vi "LINC Register Packet.vi"(4 "alternate data names (empty)":string[](array[string]), 5 "ID":i32=-1, 6 "alternate packet names (empty)":string[](array[string]), 7 "single packet (F)":bool, 8 "error in (no error)":errorcluster, 9 "type (CMD)":enum16{"CMD", "TLM", "CMD_HDR", "TLM_HDR"}(ring), 10 "controls":refnum<vi>[](array[refnum]), 11 "LINC session":refnum<class "LINC.lvclass">) -> (0 "error out":errorcluster, 3 "dup LINC session":refnum<class "LINC.lvclass">)   [LabVIEW 2018, in "STEPkgDriver_LINC.lvlib" / "LINC.lvclass"]
uses:
  LINC.lvclass
  STEPkgDriver_LINC.lvlib
  LINC Global Mode.ctl
  LINC Config.ctl
  LINC Global Config Mode.ctl
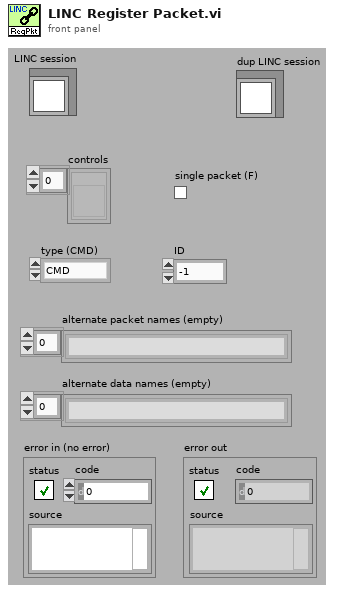
[diagram p1: front panel]
types:
  T1 = typedef "STEPkgDriver_LINC.lvlib/LINC Global Config Mode.ctl" = enum16{"INIT", "CLEAR", "SET_CMD_CB", "SET_TLM_CB", "SET_CMD_FIELDS", "SET_TLM_FIELDS", "SET_ID", "GET_CONFIG"}
  T2 = typedef "STEPkgDriver_LINC.lvlib/LINC Config.ctl" = cluster{"cmd callback":refnum<vi>, "tlm callback":refnum<vi>, "cmd ID bitoffset":i32, "cmd ID bitsize":i32, "cmd IDs":i32[], "tlm ID bitoffset":i32, "tlm ID bitsize":i32, "tlm IDs":i32[], "cmd header fields":i32, "tlm header fields":i32, "tlm header size":i32}
  T3 = typedef "STEPkgDriver_LINC.lvlib/LINC Global Mode.ctl" = enum16{"INIT", "CLEAR", "ADD_PKT_HDR", "ADD_PKT", "GET_PKT_NAMES", "GET_PKT_DESC", "GET_PKT_HDR", "GET_PKT", "SET_PKT", "SET_DATA", "SIM_EN", "SIM_DS"}
  T4 = typedef "STEPkgDriver_LINC.lvlib/LINC Format Prototype.ctl" = cluster{"type":string, "bit offset":i32, "bit size":i32, "format":string, "unit":string, "description":string, "state values":i64[], "states":string[], "max":string, "min":string, "default":string, "array":bool, "bit element size":i32, "poly bound":dbl[], "poly scale":cluster{"coefficients":dbl[]}[], "labview size":i32, "simulate":bool, "ID":bool, "required":bool}
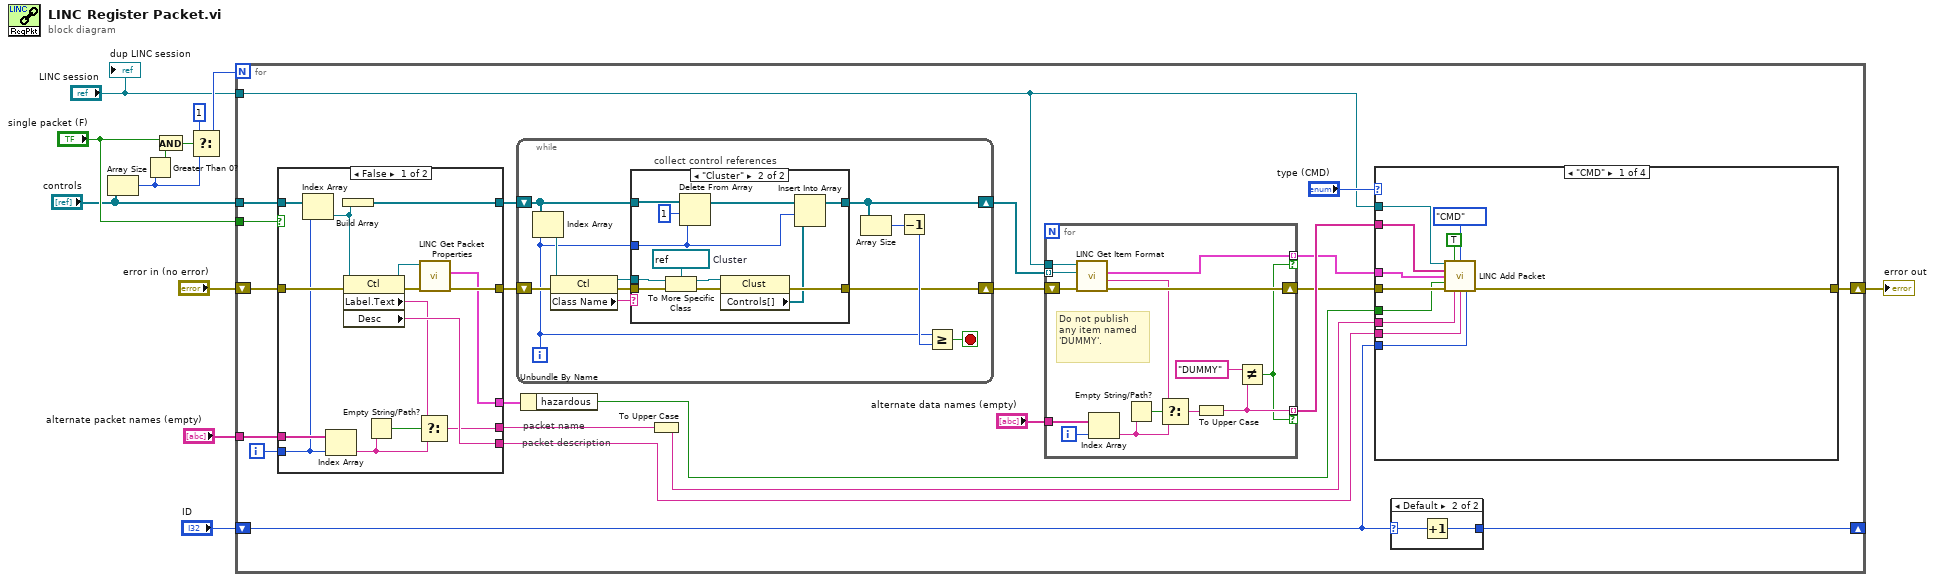
[diagram p0: block diagram]
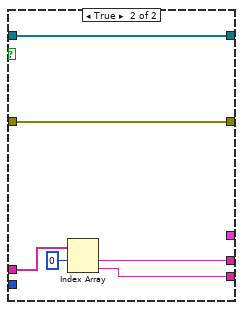
[diagram p3: hidden frame]
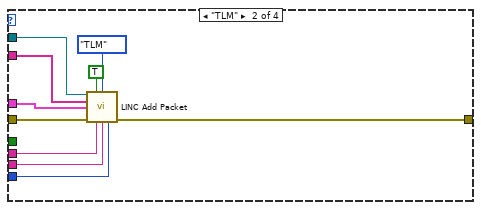
[diagram p4: hidden frame]
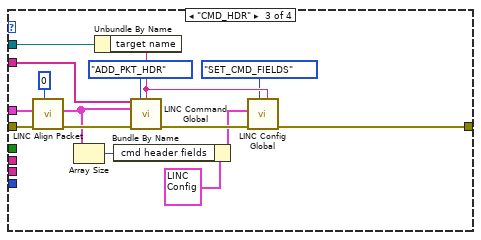
[diagram p5: hidden frame]
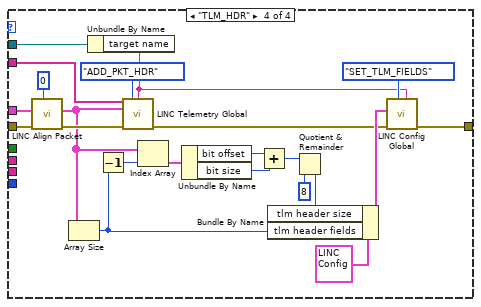
[diagram p6: hidden frame]
diagram:
  n1 = Array Size(array="controls") -> (size(s)=w8:i32)
  n2 = Greater Than 0?(x=w8) -> (x > 0?=w6:bool)
  n3 = And(x="single packet (F)", y=w6) -> (x .and. y?=w5:bool)
  n4 = Select(t=1, s=w5, f=w8) -> (s? t:f=w10:i32)
  n5 = for {
    N: w10 -> [_]
    tunnel: "controls" -> [w25]
    shift-right: [w29] -> w12
    shift-left: "error in (no error)" -> [w33]
    tunnel: "alternate packet names (empty)" -> [w28]
    tunnel: "single packet (F)" -> [w23]
    tunnel: "LINC session" -> [w15]
    shift-right: [w19] -> _
    shift-left: "ID" -> [w18]
    i -> [w24]
    # "packet description"
    # "packet name"
    n6 = case shown="False" w23 {
      tunnel: [w53 w59] -> w34
      tunnel: w33 -> [w52 w55]
      tunnel: [w41 w55] -> w21
      tunnel: [w51 w54] -> w32
      tunnel: w28 -> [w50 w58]
      tunnel: [w47 w56] -> w27
      tunnel: w25 -> [w46 w59]
      tunnel: w24 -> [w45 _]
      tunnel: [w39 _] -> w14
      frame False {
        n7 = Index Array(array=w46, index=w45) -> (element=w44:refnum<vi>)
        n8 = Index Array(array=w50, index=w45) -> (element=w48:string)
        n9 = Build Array(w44) -> (w53:refnum<vi>[])
        n10 = property class="Ctl"(reference=w44, error in=w52) -> (reference out=w40:refnum<vi>, error out=w42:errorcluster, "Label.Text"=w43:string, "Desc"=w51:string)
        n11 = Empty String/Path?(string/path=w48) -> (empty?=w49:bool)
        n12 = Select(t=w43, s=w49, f=w48) -> (s? t:f=w47:string)
        n13 = call "LINC Get Packet Properties.vi"("error in (no error)"=w42, "control reference"=w40) -> ("error out"=w41:errorcluster, "properties"=w39:cluster{"hazardous":bool})  [unwired: 8 in]
      }
      frame True {
        n14 = Index Array(array=w58, index #1=0 ("index")) -> (element #1=w56:string, element #2=w54:string)  [unwired: 1 in]
      }
    }
    n15 = while {
      shift-right: [w139] -> w20
      shift-left: w21 -> [w134]
      shift-right: [w140] -> w35
      shift-left: w34 -> [w141]
      i -> [w132]
      stop <- w138 stop-if-true
      # "collect control references"
      n16 = Index Array(array=w141, index=w132) -> (element=w133:refnum<vi>)
      n17 = property class="Ctl"(reference=w133, error in=w134) -> (reference out=w135:refnum<vi>, error out=w136:errorcluster, "Class Name"=w137:string)
      n18 = case shown="\"Cluster\"" w137 {
        tunnel: w136 -> [w145 w156]
        tunnel: w135 -> [_ w157]
        tunnel: w141 -> [w144 w149]
        tunnel: [w145 w152] -> w139
        tunnel: [w144 w151] -> w140
        tunnel: w132 -> [_ w146]
        frame Default {
        }
        frame "Cluster" {
          w153 = refnum<vi> refnum  # Cluster
          n19 = To More Specific Class(target class=w153, reference=w157, error in=w156) -> (specific class reference=w154:refnum<vi>, error out=w155:errorcluster)
          n20 = Delete From Array(array=w149, length=1, index=w146) -> (array with subset deleted=w148:refnum<vi>[])  [unwired: 1 out]
          n21 = property class="Clust"(reference=w154, error in=w155) -> (error out=w152:errorcluster, "Controls[]"=w150:refnum<vi>[])  [unwired: 1 out]
          n22 = Insert Into Array(array=w148, index=w146, new element=w150) -> (w151:refnum<vi>[])
        }
      }
      n23 = Array Size(array=w140) -> (size(s)=w143:i32)
      n24 = Decrement(x=w143) -> (x-1=w142:i32)
      n25 = Greater Or Equal?(x=w132, y=w142) -> (x >= y?=w138:bool)
    }
    n26 = Unbundle By Name(w14) -> ("hazardous"=w13:bool)
    n27 = To Upper Case(1:w27) -> (0:w16:string)
    n28 = for {
      tunnel: w35 -> [w124] mode=indexing
      tunnel: [w121] -> w26 mode=indexing if=w118
      shift-right: [w125] -> w30
      shift-left: w20 -> [w126]
      tunnel: [w120] -> w31 mode=indexing if=w118
      tunnel: "alternate data names (empty)" -> [w129]
      tunnel: w15 -> [w123]
      i -> [w128]
      # "Do not publish any item named 'DUMMY'."
      n29 = call "LINC Get Item Format.vi"("error in (no error)"=w126, "control reference"=w124, "LINC session"=w123) -> ("error out"=w125:errorcluster, "item name"=w122:string, "item format"=w121:T4)  [unwired: 6 in]
      n30 = Index Array(array=w129, index=w128) -> (element=w131:string)
      n31 = Empty String/Path?(string/path=w131) -> (empty?=w130:bool)
      n32 = Select(t=w122, s=w130, f=w131) -> (s? t:f=w127:string)
      n33 = To Upper Case(1:w127) -> (0:w120:string)
      n34 = Not Equal?(x="DUMMY", y=w120) -> (x != y?=w118:bool)
    }
    n35 = case shown="\"CMD\"" "type (CMD)" {
      tunnel: [w70 w80 w86 w105] -> w29
      tunnel: w15 -> [w68 w78 w90 w112]
      tunnel: w16 -> [w63 w73 _ _]
      tunnel: w32 -> [w62 w72 _ _]
      tunnel: w26 -> [w65 w74 w93 w114]
      tunnel: w31 -> [w69 w76 w91 w113]
      tunnel: w30 -> [w64 w75 w95 w116]
      tunnel: w18 -> [w61 w71 _ _]
      tunnel: w13 -> [w60 _ _ _]
      frame "CMD" {
        n36 = call "LINC Add Packet.vi"("LINC session"=w68, "add header (F)"=TRUE, "type (CMD)"=enum16{"CMD", "TLM"}."CMD", "item names in"=w69, "item formats in"=w65, "hazardous"=w60, "e rror in (no error)"=w64, "packet name"=w63, "packet description"=w62, "ID"=w61) -> ("error out"=w70:errorcluster)  [unwired: 4 in, 1 out]
      }
      frame "TLM" {
        n37 = call "LINC Add Packet.vi"("LINC session"=w78, "add header (F)"=TRUE, "type (CMD)"=enum16{"CMD", "TLM"}."TLM", "item names in"=w76, "item formats in"=w74, "e rror in (no error)"=w75, "packet name"=w73, "packet description"=w72, "ID"=w71) -> ("error out"=w80:errorcluster)  [unwired: 5 in, 1 out]
      }
      frame "CMD_HDR" {
        n38 = call "LINC Align Packet.vi"("initial offset"=0, "error in (no error)"=w95, "item formats in"=w93) -> ("error out"=w94:errorcluster, "item formats out"=w88:T4[])  [unwired: 7 in]
        n39 = Array Size(array=w88) -> (size(s)=w83:i32)
        n40 = Unbundle By Name(w90) -> ("target name"=w85:string)
        n41 = Bundle By Name(cluster=T2 {"cmd callback"=refnum, "tlm callback"=refnum, "cmd ID bitoffset"=0, "cmd ID bitsize"=0, "cmd IDs"=[], "tlm ID bitoffset"=0, "tlm ID bitsize"=0, "tlm IDs"=[], "cmd header fields"=0, "tlm header fields"=0, "tlm header size"=0} ("config in"), "cmd header fields"=w83) -> (w82:T2)
        n42 = call "LINC Command Global.vi"("item names in"=w91, "mode"=LINC_Global_Mode."ADD_PKT_HDR", "target name"=w85, "item formats in"=w88, "error in (no error)"=w94) -> ("error out"=w87:errorcluster)  [unwired: 6 in, 4 out]
        n43 = call "LINC Config Global.vi"("target name"=w85, "mode"=LINC_Global_Config_Mode."SET_CMD_FIELDS", "error in (no error)"=w87, "config in"=w82) -> ("error out"=w86:errorcluster)  [unwired: 6 in, 1 out]
      }
      frame "TLM_HDR" {
        n44 = call "LINC Align Packet.vi"("initial offset"=0, "error in (no error)"=w116, "item formats in"=w114) -> ("error out"=w115:errorcluster, "item formats out"=w103:T4[])  [unwired: 7 in]
        n45 = Array Size(array=w103) -> (size(s)=w104:i32)
        n46 = Unbundle By Name(w112) -> ("target name"=w106:string)
        n47 = Decrement(x=w104) -> (x-1=w102:i32)
        n48 = call "LINC Telemetry Global.vi"("item names in"=w113, "mode"=LINC_Global_Mode."ADD_PKT_HDR", "target name"=w106, "item formats in"=w103, "error in (no error)"=w115) -> ("error out"=w107:errorcluster)  [unwired: 6 in, 4 out]
        n49 = Index Array(array=w103, index=w102) -> (element=w101:T4)
        n50 = Unbundle By Name(w101) -> ("bit offset"=w100:i32, "bit size"=w99:i32)
        n51 = Add(x=w100, y=w99) -> (x+y=w98:i32)
        n52 = Quotient & Remainder(x=w98, y=8) -> (floor(x/y)=w96:i32)  [unwired: 1 out]
        n53 = Bundle By Name(cluster=T2 {"cmd callback"=refnum, "tlm callback"=refnum, "cmd ID bitoffset"=0, "cmd ID bitsize"=0, "cmd IDs"=[], "tlm ID bitoffset"=0, "tlm ID bitsize"=0, "tlm IDs"=[], "cmd header fields"=0, "tlm header fields"=0, "tlm header size"=0} ("config in"), "tlm header size"=w96, "tlm header fields"=w104) -> (w109:T2)
        n54 = call "LINC Config Global.vi"("target name"=w106, "mode"=LINC_Global_Config_Mode."SET_TLM_FIELDS", "error in (no error)"=w107, "config in"=w109) -> ("error out"=w105:errorcluster)  [unwired: 6 in, 1 out]
      }
    }
    n55 = case shown="Default" w18 {
      selector: w18 -> [w36 w37]
      tunnel: [w36 w38] -> w19
      frame -1 {
      }
      frame Default {
        n56 = Increment(x=w37) -> (x+1=w38:i32)
      }
    }
  }
  "error out" <- w12
  "dup LINC session" <- "LINC session"
